vi "Avg Data Read.vi"(4 "error in (no error)":errorcluster, 6 "Container State":T3, 7 "Display State In":T2 {"Time_data" format="%<%.3X>T"}) -> (0 "error out":errorcluster, 2 "Value":T1(array[cluster]), 3 "Display State Out":T2 {"Time_data" format="%<%.3X>T"})   [LabVIEW 2015, in "2D Buffer Display.xctl"]
uses:
  2D Buffer Display.xctl
  <vilib>/_xctls/Container State.ctl
  Graph_State.ctl
  <vilib>/_xctls/XControlSupport.lvlib
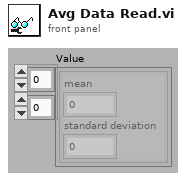
[diagram p1: front panel]
types:
  T1 = cluster{"mean":dbl, "standard deviation":dbl}[][]
  T2 = typedef "2D Buffer Display.xctl/Graph_State.ctl" = cluster{"History":u16, "Time_data":timestamp[], "Data_Out":sgl[][][], "Channels":bool[], "Variable":bool[], "Variable Tags":string[], "Channel Tags":string[], "Plot Details":cluster{"Name":string, "Line Width":u8, "Line Style":u8, "Color":u32}[], "Y-Axis Labels":string[], "Avg Data":cluster{"mean":dbl, "standard deviation":dbl}[][]}
  T3 = typedef "XControlSupport.lvlib/Container State.ctl" = cluster{"Indicator?":bool, "Run Mode?":bool, " Refnum":refnum<vi>}
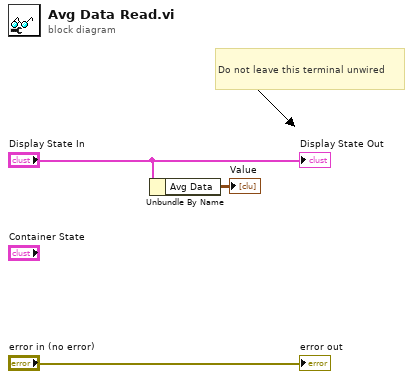
[diagram p0: block diagram]
diagram:
  # "Do not leave this terminal unwired"
  n1 = Unbundle By Name("Display State In") -> ("Avg Data"=→"Value":T1)
  "error out" <- "error in (no error)"
  "Display State Out" <- "Display State In"
